vi "TPNT_AddDevice.vi"(6 "deflogsep":string="blank", 8 "error in (no error)":errorcluster, 9 "name":string, 10 "arguments":string, 11 "Object Refnum In":T6) -> (0 "error out":errorcluster, 3 "Data Refnum out":T6)   [LabVIEW 2016]
uses:
  TPNT_Refnum.ctl
  TPNT_DeviceTPs.ctl
  TPNT_TP.ctl
  TPNT_Limits.ctl
  TPNT_Samples.ctl
  TPNT_Log.ctl
panel:
  in  "device":T1={"device"="", "devupdate"=0.0, "next_update"=0, "devinterface"="", "TPs"=[], "Alarms"=TRUE, "monitor"=TRUE, "log sep"=""} {"TPs"."Log"."updaterate" format="%.2f"; "TPs"."Samples"."Values" format="%.2f"; "TPs"."Samples"."samples" min=1 step=1; "TPs"."Limits"."Nominal" format="%.2f"; "TPs"."Limits"."Upper" format="%.2f"; "TPs"."Limits"."Lower" format="%.2f"; "TPs"."update_rate" format="%.2f"; "devupdate" format="%.2f"}
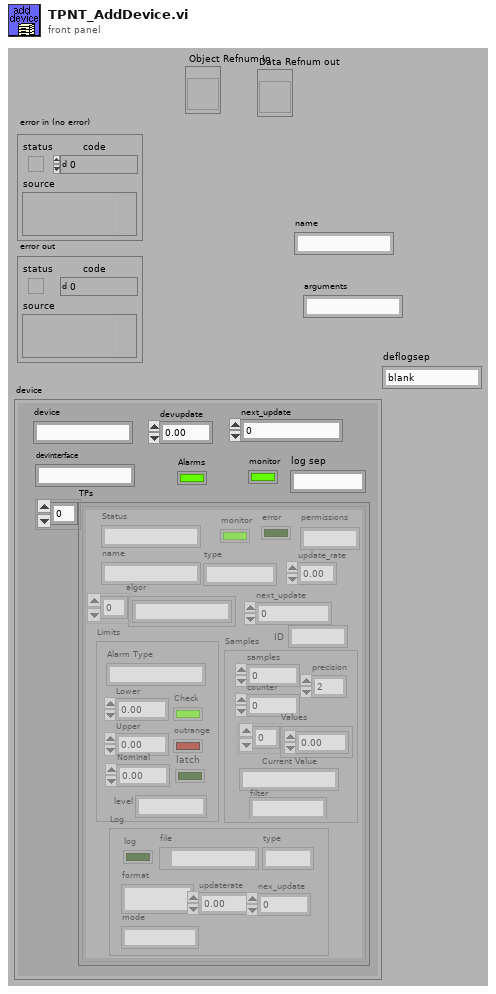
[diagram p1: front panel]
types:
  T1 = typedef "TPNT_DeviceTPs.ctl" = cluster{"device":string, "devupdate":dbl, "next_update":u32, "devinterface":string, "TPs":T2[], "Alarms":bool, "monitor":bool, "log sep":string}
  T2 = typedef "TPNT_TP.ctl" = cluster{"name":string, "type":string, "algor":string[], "update_rate":sgl, "Limits":T3, "Samples":T4, "next_update":u32, "Status":string, "monitor":bool, "error":bool, "Log":T5, "permissions":string, "ID":string}
  T3 = typedef "TPNT_Limits.ctl" = cluster{"Alarm Type":string, "Lower ":dbl, "Upper":dbl, "Nominal":dbl, "outrange":bool, "Check":bool, "latch":bool, "level":string}
  T4 = typedef "TPNT_Samples.ctl" = cluster{"samples":i32, "counter":i32, "Values":dbl[], "Current Value":string, "filter":string, "precision":u8}
  T5 = typedef "TPNT_Log.ctl" = cluster{"log":bool, "file":path, "type":string, "format":string, "updaterate":dbl, "nex_update":u32, "mode":string}
  T6 = typedef "TPNT_Refnum.ctl" = refnum<vi>
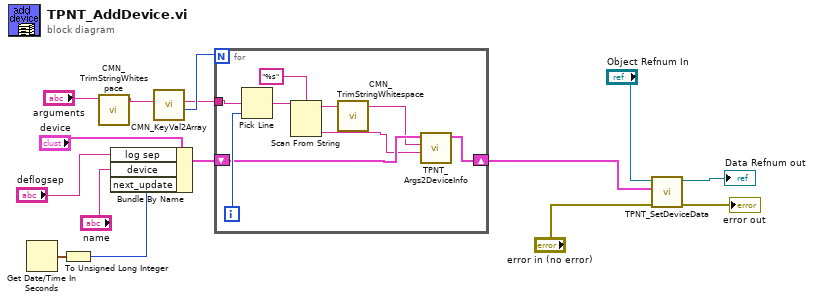
[diagram p0: block diagram]
diagram:
  n1 = Get Date/Time In Seconds() -> (seconds since 1Jan1904=w2:timestamp)
  n2 = To Unsigned Long Integer(number=w2) -> (unsigned 32bit integer=w1:u32)
  n3 = call "CMN_TrimStringWhitespace.vi"("string"="arguments") -> ("trimmed string"=w10:string)  [unwired: 1 in, 8 out]
  n4 = Bundle By Name(cluster="device", "log sep"="deflogsep", "device"="name", "next_update"=w1) -> (w6:T1)
  n5 = call "CMN_KeyVal2Array.vi"("command in"=w10) -> ("number of commands"=w13:i32, "commands out"=w12:string)  [unwired: 2 in, 6 out]
  n6 = for {
    N: w13 -> [_]
    tunnel: w12 -> [w24]
    shift-right: [w18] -> w9
    shift-left: w6 -> [w19]
    i -> [w23]
    n7 = Pick Line(multi-line string=w24, line index=w23) -> (output string=w22:string)  [unwired: 1 out]
    n8 = Scan From String(format string="%s", input string=w22) -> (remaining string=w20:string, output 1=w16:string)  [unwired: 2 in, 3 out]
    n9 = call "CMN_TrimStringWhitespace.vi"("string"=w20) -> ("trimmed string"=w17:string)  [unwired: 1 in, 8 out]
    n10 = call "TPNT_Args2DeviceInfo.vi"("key"=w16, "value"=w17, "Device IN"=w19) -> ("Device OUT"=w18:T1)  [unwired: 8 out]
  }
  n11 = call "TPNT_SetDeviceData.vi"("error in (no error)"="error in (no error)", "Object Data In"=w9, "Object Refnum In"="Object Refnum In") -> ("error out"=→"error out":errorcluster, "Data Refnum out"=→"Data Refnum out":T6)  [unwired: 7 out]
